vi "XYStage.UpdatedNamedPosition.vi"(8 "error in (no error)":errorcluster, 10 "NewNamedPosition":string, 11 "XYStage":refnum<class "XYStage.lvclass">) -> (0 "error out":errorcluster, 3 "XYStage out":refnum<class "XYStage.lvclass">)   [LabVIEW 2019, in "XYStage.lvclass"]
doc: "---------------------------------------------------------------\nJKI State Machine Objects™\nhttp://jki.net/state-machine-objects/\nCopyright (C) 2005-2015, JKI <info@jki.net>\nALL RIGHTS RESERVEDJKI State Machine Objects (SMO) 1.0.0.4\nJKI - JKI\nCopyright (c) 2015, JKI"
uses:
  XYStage.lvclass
panel:
  # "For instructions on how to use the JKI State Machine Objects, examples and video tutorials, visit:\nhttp://jki.net/state-machine-objects/\n\nJKI State Machine Objects™\nhttp://jki.net/state-machine-objects/\nCopyright (C) 2005-2015, JKI <info@jki.net>\nALL RIGHTS RESERVED"
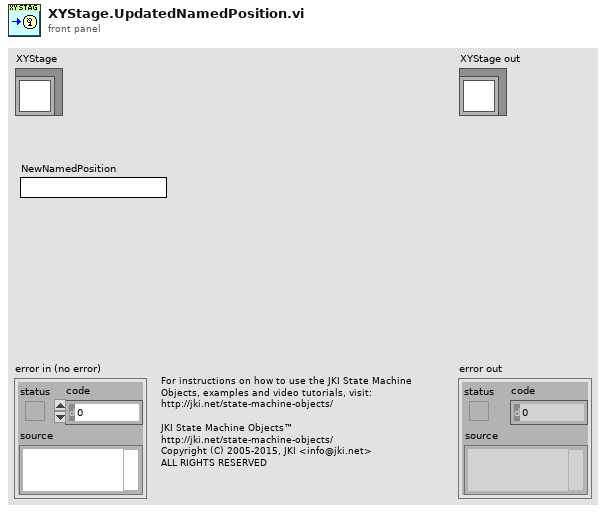
[diagram p1: front panel]
types:
  T1 = typedef "XYStage.lvclass/PrivateData--Ref.ctl" = refnum<data-value>
  T2 = typedef "XYStage.lvclass/PrivateData--Cluster.ctl" = cluster{"Dependencies":T3, "Public Events":T4, "Protected Events":T5, "Private Events":T6, "Configuration":T7, "Target":T8, "Move Parameters":T11}
  T3 = typedef "XYStage.lvclass/Dependencies--Cluster.ctl" = cluster{"Positions":refnum<class "SMO.Dictionary.Variant.lvclass">}
  T4 = typedef "XYStage.lvclass/PublicEvents--Cluster.ctl" = cluster{"MoveComplete":refnum<user-event>, "NewPosition":refnum<user-event>, "UpdatedNamedPosition":refnum<user-event>, "MoveStarted":refnum<user-event>}
  T5 = typedef "XYStage.lvclass/ProtectedEvents--Cluster.ctl" = cluster{"API_Template":refnum<user-event>}
  T6 = typedef "XYStage.lvclass/PrivateEvents--Cluster.ctl" = cluster{"MoveAbsolute":refnum<user-event>, "MoveRelative":refnum<user-event>, "MoveToNamedPosition":refnum<user-event>, "StorePosition":refnum<user-event>, "Home":refnum<user-event>}
  T7 = typedef "XYStage.lvclass/Configuration--Cluster.ctl" = cluster{"Real-World Units":string, "Counts per Unit":dbl}
  T8 = typedef "XYStage.lvclass/TargetPositions--Cluster.ctl" = cluster{"Coords":T9, "Counts":T10}
  T9 = typedef "XYStage.lvclass/(real)Coords--Cluster.ctl" = cluster{"X":dbl, "Y":dbl}
  T10 = typedef "XYStage.lvclass/(counts)Coords--Cluster.ctl" = cluster{"X":i32, "Y":i32}
  T11 = typedef "XYStage.lvclass/MoveParameters--Cluster.ctl" = cluster{"Velocity (units/s)":dbl, "Acceleration (units/s^2)":dbl}
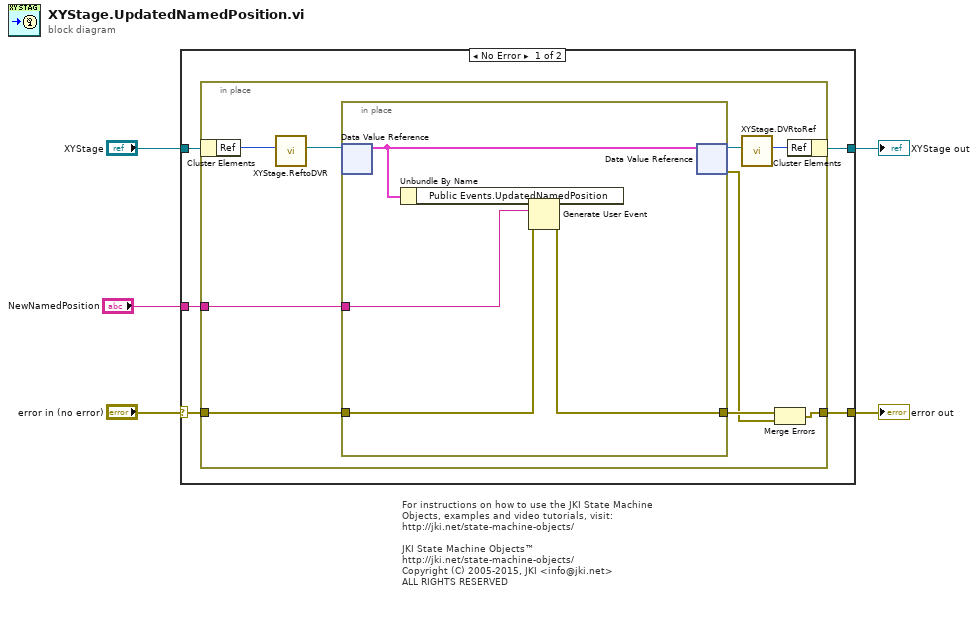
[diagram p0: block diagram]
diagram:
  # "For instructions on how to use the JKI State Machine Objects, examples and video tutorials, visit:\nhttp://jki.net/state-machine-objects/\n\nJKI State Machine Objects™\nhttp://jki.net/state-machine-objects/\nCopyright (C) 2005-2015, JKI <info@jki.net>\nALL RIGHTS RESERVED"
  n1 = case shown="No Error" "error in (no error)" {
    selector: "error in (no error)" -> [w8 w26]
    tunnel: [w7 w26] -> w4
    tunnel: [w9 w25] -> w5
    tunnel: "XYStage" -> [w10 w25]
    tunnel: "NewNamedPosition" -> [w6 _]
    frame No Error {
      n2 = in-place {
        in-place-border: w8 -> [w19]
        in-place-border: [w16] -> w7
        in-place-border: w6 -> [w13]
        n3 = in-place-cluster #1(w10) -> ("Ref"=w15:u32)
        n4 = call "XYStage.ReftoDVR.vi"("Ref"=w15) -> ("Ref"=w12:T1)  [unwired: 10 in]
        n5 = in-place {
          in-place-border: w19 -> [w23]
          in-place-border: [w22] -> w18
          in-place-border: w13 -> [w21]
          n6 = in-place-dvr #2(w12) -> (w20:T2)  [unwired: 1 out]
          n7 = Unbundle By Name(w20) -> ("Public Events.UpdatedNamedPosition"=w24:refnum<user-event>)
          n8 = Generate User Event(user event=w24, event data cluster=w21, error in=w23) -> (error out=w22:errorcluster)  [unwired: 1 in, 1 out]
          n9 = in-place-dvr #2(w20) -> (w14:T1, w17:errorcluster)
        }
        n10 = call "XYStage.DVRtoRef.vi"("Ref"=w14) -> ("Ref"=w11:u32)  [unwired: 10 in]
        n11 = Merge Errors(w18, w17) -> (w16:errorcluster)
        n12 = in-place-cluster #1("Ref"=w11) -> (w9:refnum<class "XYStage.lvclass">)
      }
    }
    frame Error {
    }
  }
  "error out" <- w4
  "XYStage out" <- w5
